vi "Boolean to On or Off.vi"(4 "Boolean":bool) -> (0 "lowercase":string, 1 "UPPERCASE":string, 2 "Capitalized":string)   [LabVIEW 2020, in "Utilities.lvlib"]
doc: "Converts a boolean to either \"On\" or \"Off\". The string is returned capitalized, in all uppercase, and in all lowercase."
uses:
  Utilities.lvlib
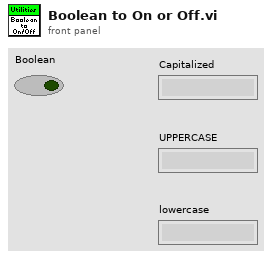
[diagram p1: front panel]
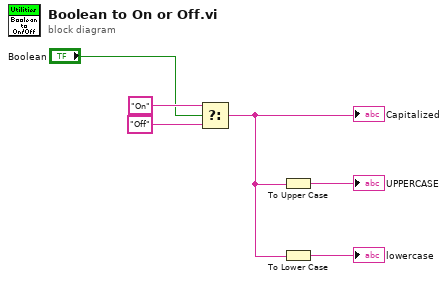
[diagram p0: block diagram]
diagram:
  n1 = Select(t="On", s="Boolean", f="Off") -> (s? t:f=w1:string)
  "Capitalized" <- w1
  n2 = To Upper Case(1:w1) -> (0:→"UPPERCASE":string)
  n3 = To Lower Case(string=w1) -> (all lower case string=→"lowercase":string)
